vi "LoopClockDeamon.vi"(6 "Instance":i32, 10 "milliseconds to wait":u32=200, 11 "VI Refnum":refnum<vi>) -> ()   [LabVIEW 2017, in "Communication.lvlib"]
uses:
  Communication.lvlib
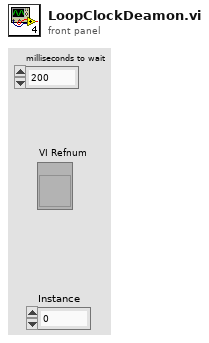
[diagram p1: front panel]
types:
  T1 = enum32{"Bad", "Idle", "Run top level", "Running"}
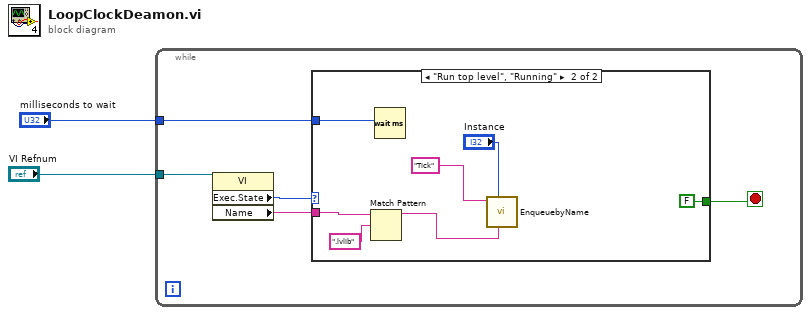
[diagram p0: block diagram]
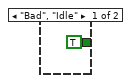
[diagram p2: hidden frame]
diagram:
  n1 = while {
    tunnel: "VI Refnum" -> [w7]
    tunnel: "milliseconds to wait" -> [w5]
    stop <- w4 stop-if-true
    n2 = property class="VI"(reference=w7) -> ("Exec.State"=w6:T1, "Name"=w3:string)  [unwired: 1 in, 2 out]
    n3 = case shown="\"Run top level\", \"Running\"" w6 {
      tunnel: w5 -> [_ w15]
      tunnel: [TRUE FALSE] -> w4
      tunnel: w3 -> [_ w12]
      frame "Bad", "Idle" {
      }
      frame "Run top level", "Running" {
        n4 = Match Pattern(string=w12, regular expression=".lvlib") -> (before substring=w10:string)  [unwired: 1 in, 3 out]
        n5 = Wait (ms)(milliseconds to wait=w15) -> ()  [unwired: 1 out]
        n6 = call "EnqueuebyName.vi"("Loop Name"=w10, "Instance"="Instance", "Msg"="Tick") -> ()  [unwired: 8 in, 1 out]
      }
    }
  }
